vi "Write Action Success.vi"(8 "error in (no error)":errorcluster, 10 "Action Success?":bool, 11 "Report Data in":refnum<class "Report Data.lvclass">) -> (0 "error out":errorcluster, 3 "Report Data out":refnum<class "Report Data.lvclass">)   [LabVIEW 2020]
uses:
  Report Data.lvclass
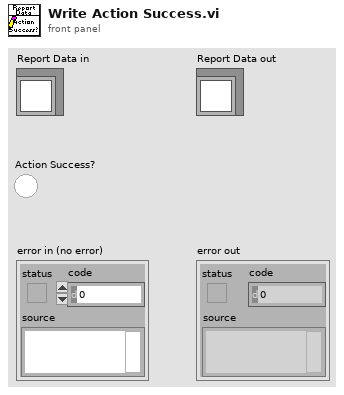
[diagram p1: front panel]
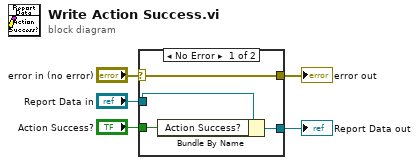
[diagram p0: block diagram]
diagram:
  n1 = case shown="No Error" "error in (no error)" {
    selector: "error in (no error)" -> [w9 w10]
    tunnel: [w9 w10] -> w4
    tunnel: [w7 w11] -> w2
    tunnel: "Report Data in" -> [w8 w11]
    tunnel: "Action Success?" -> [w6 _]
    frame No Error {
      n2 = Bundle By Name(cluster=w8, "Action Success?"=w6) -> (w7:refnum<class "Report Data.lvclass">)
    }
    frame Error {
    }
  }
  "error out" <- w4
  "Report Data out" <- w2
